vi "Sequence Complete Event Callback.vi"(4 "Sequence Complete Event Data":refnum<user-event>, 5 "Event Data":cluster{"sender":refnum<k24>, "e":refnum<k24>}, 6 "Control Ref":refnum<k24>, 7 "Event Common Data":T1) -> ()   [LabVIEW 2020, in "NI_VS Sequence Execution Interface.lvlib"]
uses:
  <vilib>/NI VeriStand/Execution/SequenceExecutionInterface/NI_VS Sequence Execution Interface.lvlib
  NationalInstruments.VeriStand.ClientAPI
  <vilib>/NI VeriStand/Execution/SequenceExecutionInterface/Sequence Complete Event Data.ctl
  <vilib>/NI VeriStand/Execution/SequenceExecutionInterface/Data Value Ref.ctl
  NationalInstruments.VeriStand.DataTypes
  NationalInstruments.VeriStand
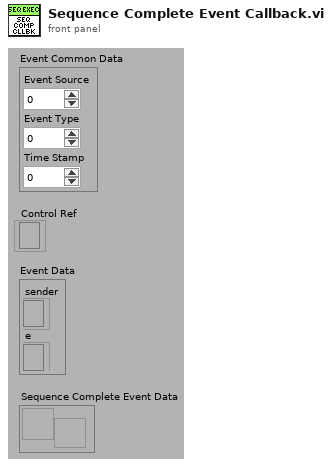
[diagram p1: front panel]
types:
  T1 = cluster{"Event Source":i32, "Event Type":u32, "Time Stamp":u32}
  T2 = typedef "NI_VS Sequence Execution Interface.lvlib/Sequence Complete Event Data.ctl" = cluster{"Sequence Name":string, "Return Value":T3, "Aborted":bool, "Error":errorcluster}
  T3 = typedef "NI_VS Sequence Execution Interface.lvlib/Data Value Ref.ctl" = refnum<k24>
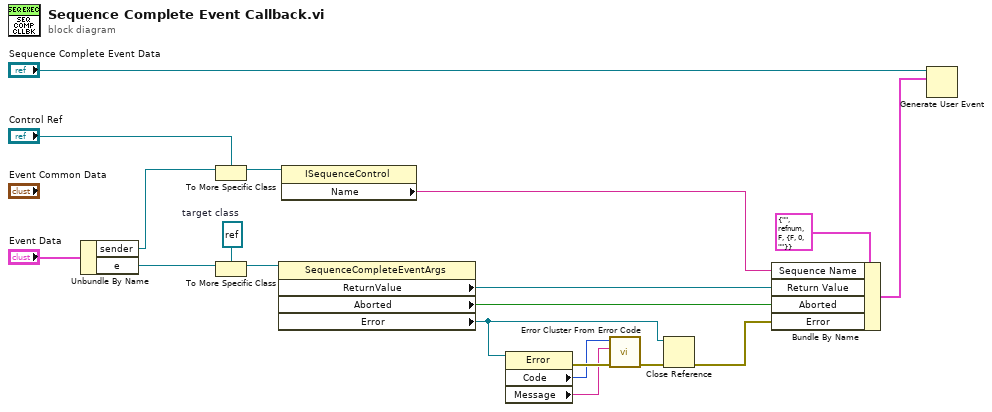
[diagram p0: block diagram]
diagram:
  w18 = refnum<k24> refnum  # target class
  n1 = Unbundle By Name("Event Data") -> ("sender"=w10:refnum<k24>, "e"=w9:refnum<k24>)
  n2 = To More Specific Class(target class="Control Ref", reference=w10) -> (specific class reference=w19:refnum<k24>)  [unwired: 1 in, 1 out]
  n3 = To More Specific Class(target class=w18, reference=w9) -> (specific class reference=w17:refnum<k24>)  [unwired: 1 in, 1 out]
  n4 = property class="SequenceCompleteEventArgs"(reference=w17) -> ("ReturnValue"=w15:refnum<k24>, "Aborted"=w14:bool, "Error"=w2:refnum<k24>)  [unwired: 1 in, 2 out]
  n5 = property class="ISequenceControl"(reference=w19) -> ("Name"=w16:string)  [unwired: 1 in, 2 out]
  n6 = property class="Error"(reference=w2) -> (error out=w6:errorcluster, "Code"=w5:u32, "Message"=w4:string)  [unwired: 1 in, 1 out]
  n7 = call <vilib>:"Error Cluster From Error Code.vi"("error in (no error)"=w6, "error message (\"\")"=w4, "error code (0)"=w5) -> ("error out"=w3:errorcluster)  [unwired: 6 in]
  n8 = Close Reference(reference=w2, error in (no error)=w3) -> (error out=w1:errorcluster)
  n9 = Bundle By Name(cluster=T2 {"Sequence Name"="", "Return Value"=refnum, "Aborted"=FALSE, "Error"={"status"=FALSE, "code"=0, "source"=""}} ("Sequence Complete Event Data"), "Sequence Name"=w16, "Return Value"=w15, "Aborted"=w14, "Error"=w1) -> (w13:T2)
  n10 = Generate User Event(user event="Sequence Complete Event Data", event data cluster=w13) -> ()  [unwired: 2 in, 2 out]
